vi "Write server listener.vi"(10 "server listener":refnum<data-value>, 11 "basic HTTP handler dataset in":refnum<class "HTTPS handler dataset.lvclass">) -> (3 "basic HTTP handler dataset out":refnum<class "HTTPS handler dataset.lvclass">)   [LabVIEW 2016, in "HTTPS handler dataset.lvclass"]
uses:
  HTTPS handler dataset.lvclass
  lvlibtls/server/lvlibretls server listener.lvclass
  HTTPS handler dataset.lvclass/HTTPS handler dataset.ctl
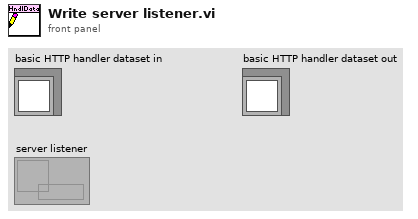
[diagram p1: front panel]
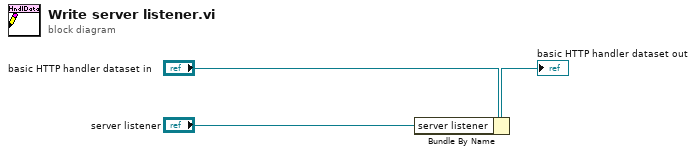
[diagram p0: block diagram]
diagram:
  n1 = Bundle By Name(cluster="basic HTTP handler dataset in", "server listener"="server listener") -> (→"basic HTTP handler dataset out":refnum<class "HTTPS handler dataset.lvclass">)
